vi "Oscillazioni.vi"(10 "y":dbl, 11 "x":dbl) -> (3 "x 2":dbl)   [LabVIEW 2018]
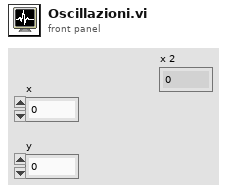
[diagram p1: front panel]
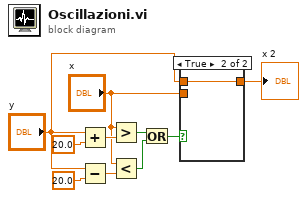
[diagram p0: block diagram]
diagram:
  n1 = Add(x="y", y=20.0) -> (x+y=w6:dbl)
  n2 = Subtract(x="y", y=20.0) -> (x-y=w8:dbl)
  n3 = Greater?(x="x", y=w6) -> (0:w10:bool)
  n4 = Less?(x="x", y=w8) -> (x < y?=w9:bool)
  n5 = Or(x=w10, y=w9) -> (x .or. y?=w4:bool)
  n6 = case shown="True" w4 {
    tunnel: [w11 w12] -> w1
    tunnel: "x" -> [w11 _]
    tunnel: "y" -> [_ w12]
    frame False {
    }
    frame True {
    }
  }
  "x 2" <- w1
